vi "Pruebas.vi"() -> ()   [LabVIEW 2017]
uses:
  EnumEstados1.ctl
panel:
  in  "Guardar en:":path
  in  "Reiniciar":bool caption="Blank Button"
  in  "Stop Button":bool
  out "Curva Corriente-Voltaje:":cluster{dbl[], "Filtered X":dbl[]}(graph)
  in  "Ok":bool
  in  "Voltaje final:":dbl
  in  "Voltaje inicial:":dbl
  in  "Paso":dbl
  # "Pruebas OLED"
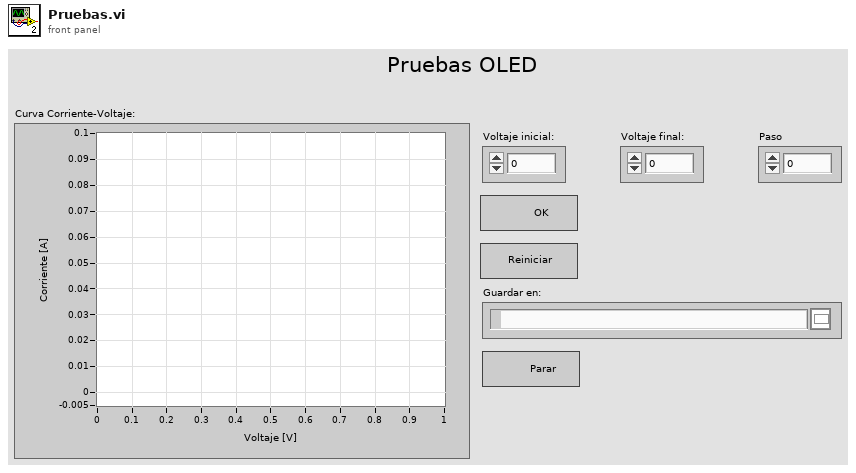
[diagram p1: front panel]
types:
  T1 = typedef "EnumEstados1.ctl" = enum16{"Inicio", "LecturaDatos", "Cierre"}
  T2 = enum16{"open", "open or create", "create or replace", "create", "open (read-only)"}
  T3 = cluster{"task out":refnum<k21>, "error out":errorcluster}
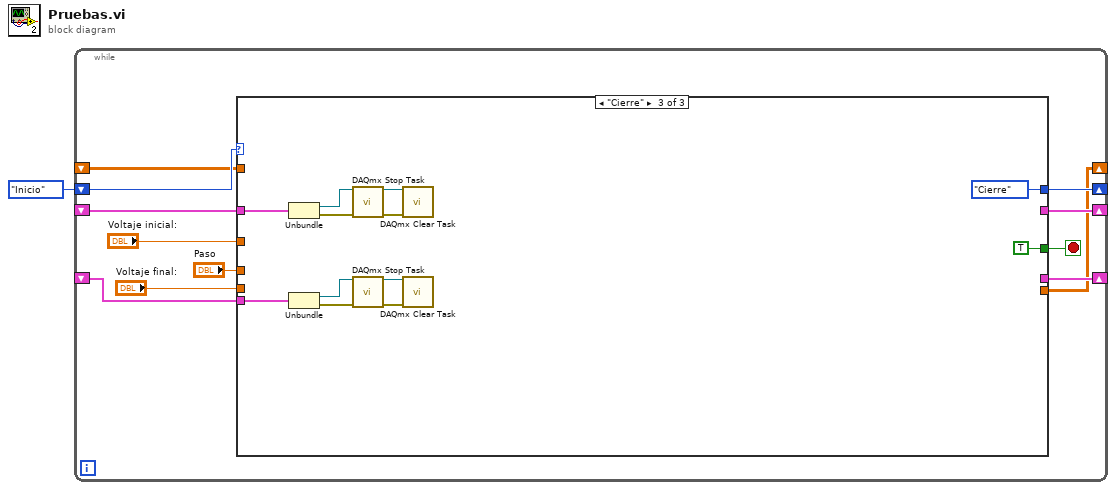
[diagram p0: block diagram]
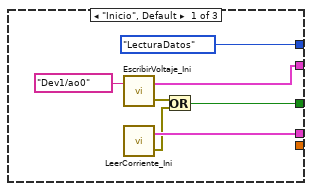
[diagram p2: hidden frame]
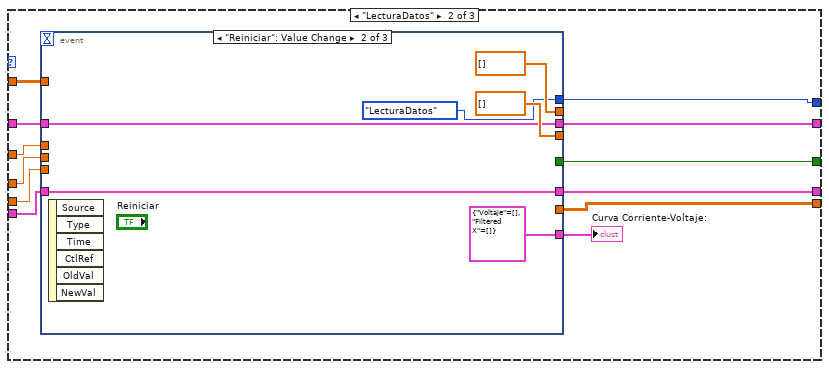
[diagram p3: hidden frame]
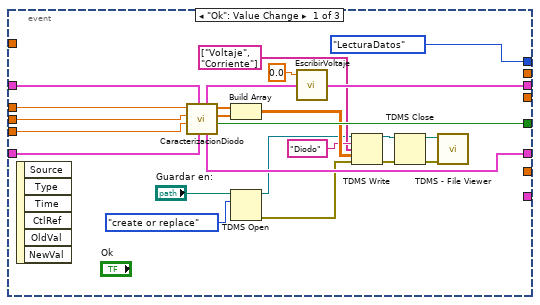
[diagram p4: hidden frame]
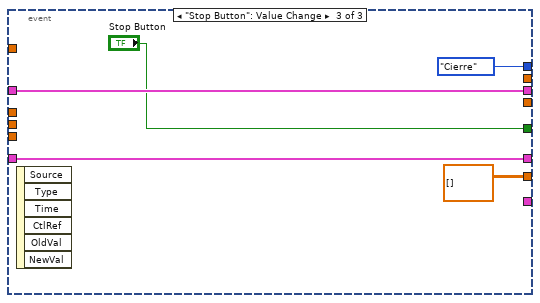
[diagram p5: hidden frame]
diagram:
  n1 = while {
    shift-right: [w5] -> _
    shift-left: EnumEstados1."Inicio" -> [w13]
    shift-right: [w9] -> _
    shift-left: _ -> [w8]
    shift-right: [w7] -> _
    shift-left: _ -> [w6]
    shift-right: [w4] -> _
    shift-left: _ -> [w3]
    stop <- w2 stop-if-true
    n2 = case shown="\"Cierre\"" w13 {
      tunnel: "Voltaje final:" -> [_ w32 _]
      tunnel: "Voltaje inicial:" -> [_ w26 _]
      tunnel: "Paso" -> [_ w27 _]
      tunnel: [w19 w30 _] -> w9
      tunnel: w8 -> [_ w31 w75]
      tunnel: [w18 w28 _] -> w7
      tunnel: w6 -> [_ w29 w74]
      tunnel: [EnumEstados1."LecturaDatos" w25 EnumEstados1."Cierre"] -> w5
      tunnel: [_ w24 _] -> w4
      tunnel: w3 -> [_ w23 _]
      tunnel: [w15 w22 TRUE] -> w2
      frame "Inicio", Default {
        n3 = call "EscribirVoltaje_Ini.vi"("physical channels"=tag "Dev1/ao0") -> ("error out"=w17:errorcluster, "cluster"=w19:T3)  [unwired: 1 in]
        n4 = call "LeerCorriente_Ini.vi"() -> ("error out"=w16:errorcluster, "output cluster"=w18:T3)  [unwired: 2 in]
        n5 = Or(x=w17, y=w16) -> (x .or. y?=w15:bool)
      }
      frame "LecturaDatos" {
        n6 = event shown="[1] \"Reiniciar\": Value Change" {
          selector: _ -> [_ _ _]
          dyn-events: _ -> [_ _ _]
          timeout: _ -> [_ _ _]
          tunnel: w32 -> [w51 _ _]
          tunnel: w31 -> [w50 w58 w67]
          tunnel: [w56 w58 w67] -> w30
          tunnel: w29 -> [w49 w57 w66]
          tunnel: [w47 w57 w66] -> w28
          tunnel: w27 -> [w52 _ _]
          tunnel: w26 -> [w53 _ _]
          tunnel: [EnumEstados1."LecturaDatos" EnumEstados1."LecturaDatos" EnumEstados1."Cierre"] -> w25
          tunnel: [_ _ dbl[][] []] -> w24
          tunnel: w23 -> [_ _ _]
          tunnel: [w46 _ "Stop Button"] -> w22
          tunnel: [_ dbl[] [] _] -> _
          tunnel: [_ dbl[] [] _] -> _
          tunnel: [_ cluster{"Voltaje":dbl[], "Filtered X":dbl[]} {"Voltaje"=[], "Filtered X"=[]} _] -> w21
          event "Ok": Value Change {
            n7 = event-data() -> ()  [unwired: 1 in, 6 out]
            n8 = call "CaracterizacionDiodo.vi"("Corriente"=w49, "Voltaje"=w50, "Voltaje final:"=w51, "Paso"=w52, "Voltaje inicial:"=w53) -> ("Error?"=w46:bool, 2:"Corriente"=w43:dbl[], 3:"Voltaje"=w44:dbl[], 4:"Corriente"=w47:T3, 5:"Voltaje"=w48:T3)  [unwired: 2 in]
            n9 = Build Array(w44, w43) -> (w42:dbl[][])
            n10 = TDMS Open(10:T2."create or replace" ("operation (0:open)"), 11:"Guardar en:") -> (0:w38:errorcluster, 3:w35:refnum<k34>)  [unwired: 5 in]
            n11 = call "EscribirVoltaje.vi"("cluster"=w48, "data"=0.0) -> ("Cluster"=w56:T3)  [unwired: 1 in, 2 out]
            n12 = TDMS Write(0:w35, 5:"Diodo" ("group name in (Untitled)"), 7:string[] ["Voltaje", "Corriente"] ("channel name(s) in (Untitled)"), 9:w42, 11:w38) -> (4:w36:refnum<k34>, 15:w37:errorcluster)  [unwired: 1 in, 2 out]
            n13 = TDMS Close(8:w37, 11:w36) -> (0:w34:errorcluster, 3:w33:path)
            n14 = call <vilib>:"TDMS - File Viewer.vi"("error in (no error)"=w34, "file path"=w33) -> ()  [unwired: 4 in, 2 out]
          }
          event "Reiniciar": Value Change {
            n15 = event-data() -> ()  [unwired: 1 in, 6 out]
          }
          event "Stop Button": Value Change {
            n16 = event-data() -> ()  [unwired: 1 in, 6 out]
          }
        }
        "Curva Corriente-Voltaje:" <- w21
      }
      frame "Cierre" {
        n17 = Unbundle(w75) -> ("task out"=w73:refnum<k21>, "error out"=w72:errorcluster)
        n18 = Unbundle(w74) -> ("task out"=w71:refnum<k21>, "error out"=w70:errorcluster)
        n19 = call <vilib>:"DAQmx Stop Task.vi"("task/channels in"=w73, "error in"=w72) -> ("task out"=w79:refnum<k21>, "error out"=w78:errorcluster)  [unwired: 12 in]
        n20 = call <vilib>:"DAQmx Stop Task.vi"("task/channels in"=w71, "error in"=w70) -> ("task out"=w77:refnum<k21>, "error out"=w76:errorcluster)  [unwired: 12 in]
        n21 = call <vilib>:"DAQmx Clear Task.vi"("task in"=w79, "error in"=w78) -> ()  [unwired: 13 in, 1 out]
        n22 = call <vilib>:"DAQmx Clear Task.vi"("task in"=w77, "error in"=w76) -> ()  [unwired: 13 in, 1 out]
      }
    }
  }
